vi "Set Icon Inside Generic.vi"(8 "error in":errorcluster, 10 "Icon":refnum<class "Icon.lvclass">, 11 "Generic Refnum in":refnum<vi>) -> (0 "error out":errorcluster, 3 "Generic Refnum out":refnum<vi>)   [LabVIEW 2024, in "XNode Support.lvlib"]
doc: "Specifies the LabVIEW Icon class of a VI."
uses:
  XNode Support.lvlib
  <vilib>/LabVIEW Icon API/lv_icon/Classes/Icon/Icon.lvclass
  <vilib>/LabVIEW Icon API/LabVIEW Icon API.lvlib
  <vilib>/LabVIEW Icon API/lv_icon/lv_icon.lvlib
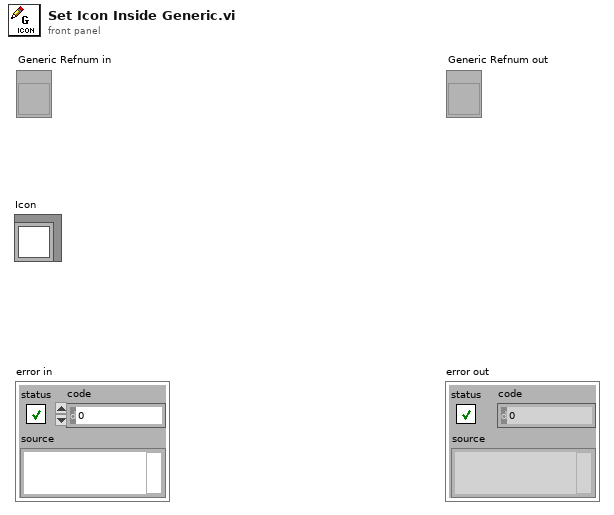
[diagram p1: front panel]
types:
  T1 = typedef "LabVIEW Icon Stored Information.ctl" = cluster{"Text Visible?":bool, "Text Opacity":u8, "Templ Visible?":bool, "Templ Opacity":u8, "Relative Path from 1 to 2":path, "Image":picture, "All User Layers":refnum<class "Layer.lvclass">[], "Body Text":T2}
  T2 = typedef "BodyText.ctl" = cluster{"Line 1 text":string, "Line 2 text":string, "Line 3 text":string, "Line 4 text":string, "Line 1 color":u32, "Line 2 color":u32, "Line 3 color":u32, "Line 4 color":u32, "Body Text Spec":cluster{"Font":T3, "Alignment":T4, "Size":u8}, "Center text vertically":bool, "Capitalize Text":bool}
  T3 = typedef "Font.ctl" = string
  T4 = typedef "Alignment.ctl" = u16
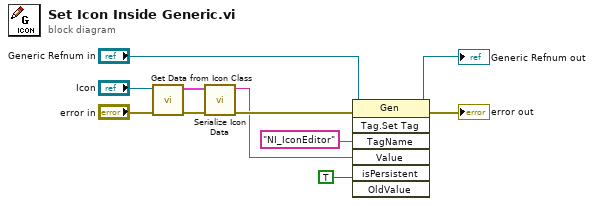
[diagram p0: block diagram]
diagram:
  n1 = call <vilib>:"Get Data from Icon Class.vi"("error in (no error)"="error in", "Icon in"="Icon") -> ("error out"=w6:errorcluster, "Icon data"=w5:T1)  [unwired: 6 in, 2 out]
  n2 = call <vilib>:"Serialize Icon Data.vi"("error in"=w6, "Icon data"=w5) -> ("error out"=w4:errorcluster, "data string"=w3:string)  [unwired: 8 in]
  n3 = invoke class="Gen" method="Tag.Set Tag"(reference="Generic Refnum in", error in=w4, "TagName"="NI_IconEditor" ("Tag Name"), "Value"=w3, "isPersistent"=TRUE ("Is Persistent")) -> (reference out=→"Generic Refnum out":refnum<vi>, error out=→"error out":errorcluster)  [unwired: 2 in, 5 out]
